vi "log_event_notifier.vi"(8 "error in":errorcluster) -> (0 "error out":errorcluster, 2 "Log event notifier":refnum<notifier>)   [LabVIEW 2012]
uses:
  log_event.ctl
panel:
  # "Get log_event notifier that is used for receiving events corresponding to state changes."
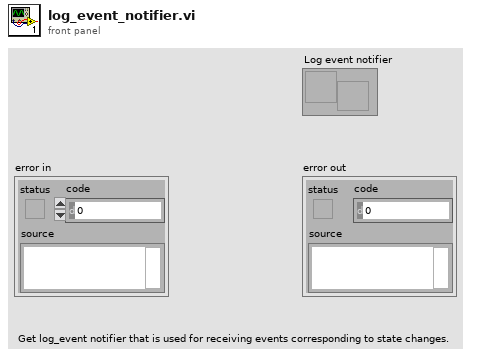
[diagram p1: front panel]
types:
  T1 = typedef "log_event.ctl" = cluster{"Facility ID":i32, "Severity":enum16{"OK", "Debug", "Warn", "Error"}, "Timestamp":timestamp, "Facility":string, "State":string, "Message":string}
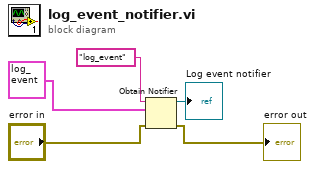
[diagram p0: block diagram]
diagram:
  n1 = Obtain Notifier(name (unnamed)="log_event", notification data type=T1 {"Facility ID"=0, "Severity"=enum."Debug", "Timestamp"=timestamp(0 s since 1904-01-01), "Facility"="", "State"="", "Message"=""} ("Log event"), error in (no error)="error in") -> (notifier out=→"Log event notifier":refnum<notifier>, error out=→"error out":errorcluster)  [unwired: 1 in, 1 out]
